vi "Check Limits.vi"(8 "error in (no error)":errorcluster, 11 "SignalWithAlarm in":refnum<class "SignalWithAlarm.lvclass">) -> (0 "error out":errorcluster, 3 "SignalWithAlarm out":refnum<class "SignalWithAlarm.lvclass">)   [LabVIEW 2016, in "SignalWithAlarm.lvclass"]
uses:
  SignalWithAlarm.lvclass
  C:/Github/LV-Class-Event-Register-Node/Signal Example/ScalarSignal Class/ScalarSignal.lvclass
  ScalarSignal Class/ScalarSignal.lvclass/ScalarSignal.ctl
  SignalWithAlarm.lvclass/SignalWithAlarm.ctl
  ScalarSignal Class/Read Data.vi
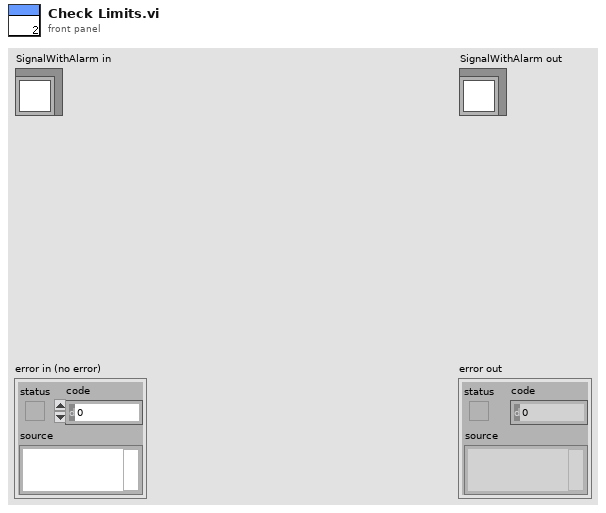
[diagram p1: front panel]
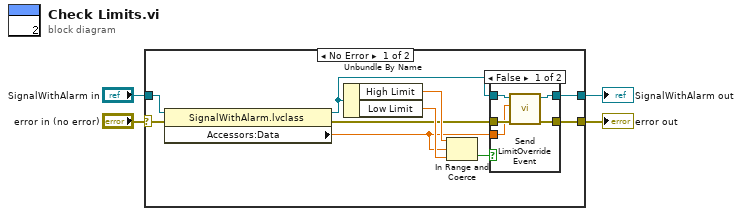
[diagram p0: block diagram]
diagram:
  n1 = case shown="No Error" "error in (no error)" {
    selector: "error in (no error)" -> [w7 w23]
    tunnel: [w9 w23] -> w3
    tunnel: [w8 w22] -> w1
    tunnel: "SignalWithAlarm in" -> [w14 w22]
    frame No Error {
      n2 = property class="SignalWithAlarm.lvclass"(reference=w14, error in=w7) -> (reference out=w11:refnum<class "SignalWithAlarm.lvclass">, error out=w6:errorcluster, "Accessors:Data"=w5:dbl)
      n3 = Unbundle By Name(w11) -> ("High Limit"=w13:dbl, "Low Limit"=w12:dbl)
      n4 = In Range and Coerce(upper limit=w13, x=w5, lower limit=w12) -> (In Range?=w10:bool)  [unwired: 1 out]
      n5 = case shown="False" w10 {
        tunnel: w11 -> [w19 w20]
        tunnel: w6 -> [w18 w21]
        tunnel: [w17 w21] -> w9
        tunnel: [w16 w20] -> w8
        tunnel: w5 -> [w15 _]
        frame False {
          n6 = call "Send LimitOverride Event.vi"("error in (no error)"=w18, "event data"=w15, "SignalWithAlarm in"=w19) -> ("error out"=w17:errorcluster, "SignalWithAlarm out"=w16:refnum<class "SignalWithAlarm.lvclass">)  [unwired: 7 in]
        }
        frame True {
        }
      }
    }
    frame Error {
    }
  }
  "error out" <- w3
  "SignalWithAlarm out" <- w1
